vi "rqcBob Close ServiceNET.vi"(8 "error in":errorcluster, 11 "rqcBob ServiceNET control":T1) -> (0 "error out":errorcluster)   [LabVIEW 2018]
uses:
  Custom Controls/rqcBob ServiceNET control.ctl
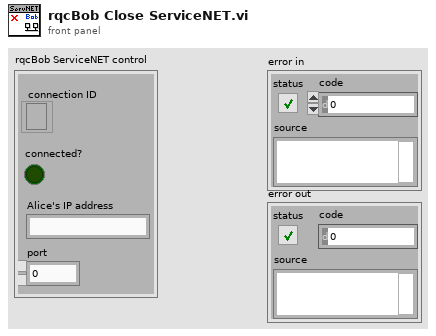
[diagram p1: front panel]
types:
  T1 = typedef "rqcBob ServiceNET control.ctl" = cluster{"connection ID":refnum<k5>, "connected?":bool, "Alice's IP address":string, "port":u16}
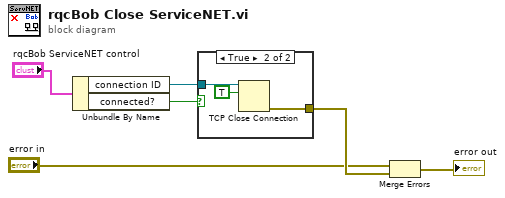
[diagram p0: block diagram]
diagram:
  n1 = Unbundle By Name("rqcBob ServiceNET control") -> ("connection ID"=w4:refnum<k5>, "connected?"=w5:bool)
  n2 = case shown="True" w5 {
    tunnel: w4 -> [_ w9]
    tunnel: [_ w8] -> w3
    frame False {
    }
    frame True {
      n3 = TCP Close Connection(connection ID=w9, abort (F)=TRUE) -> (error out=w8:errorcluster)  [unwired: 1 in, 1 out]
    }
  }
  n4 = Merge Errors("error in", w3) -> (→"error out":errorcluster)
